vi "FTW-CodeGen-EnumerateVIServerClassHierarchy.vi"(0 "Class":string="GObject", 5 "Ancestor":string="Generic", 11 "error in":errorcluster) -> (6 "Is Descendent?":bool, 15 "error out":errorcluster)   [LabVIEW 2015]
panel:
  out "VI Server Class Hierarchy":T1(array[cluster])
  # "Inputs"
  # "Outputs"
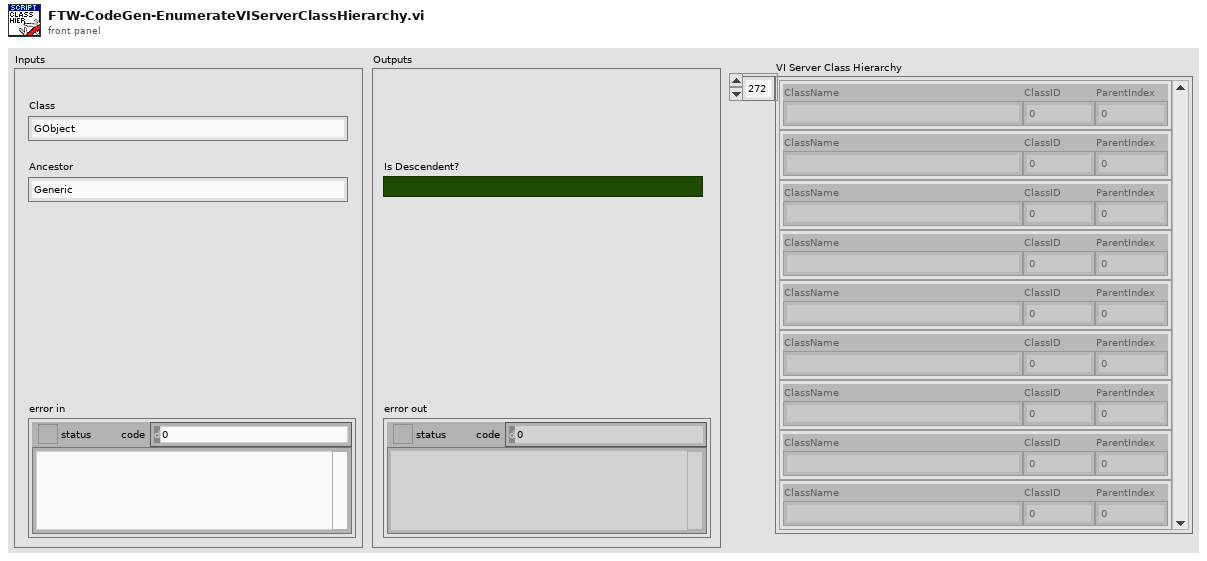
[diagram p1: front panel]
types:
  T1 = cluster{"ClassName":string, "ClassID":i32, "ParentIndex":i32}[]
  T2 = cluster{"ClassName":string, "ClassID":i32, "ParentIndex":i32}
  T3 = typedef "ASC_ArrayOfUniqueIDStringParentIDStringName.ctl" = T4[]
  T4 = typedef "ASC_UniqueIDStringParentIDStringName.ctl" = cluster{"Unique ID string":string, "Parent ID string":string, "Class Name (unlocalized)":string, "Class Name (localized)":string}
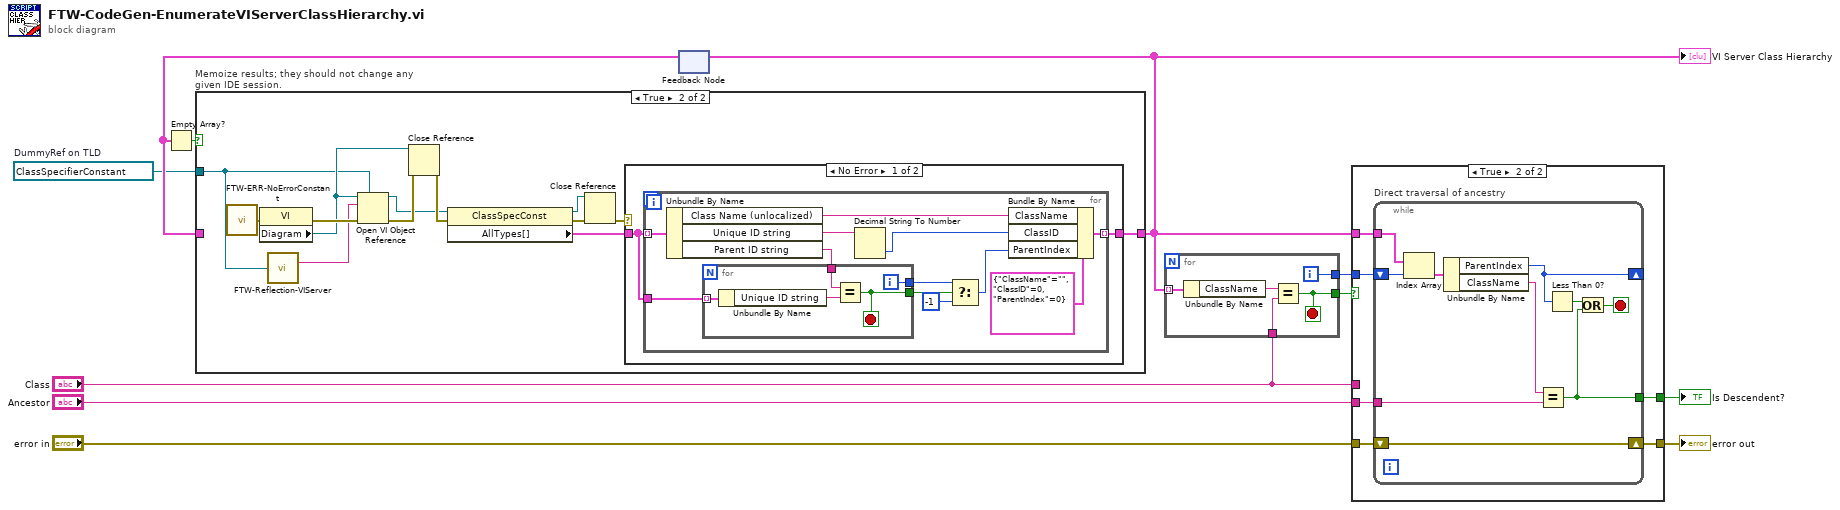
[diagram p0: block diagram]
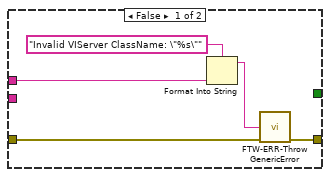
[diagram p2: hidden frame]
diagram:
  w9 = refnum<vi> refnum  # DummyRef on TLD
  n1 = feedback #1() -> (w11:T1)  [unwired: 1 in]
  n2 = Empty Array?(array=w11) -> (empty?=w10:bool)
  n3 = case "Memoize results; they should not change any given IDE session." shown="True" w10 {
    tunnel: [w12 w25] -> w4
    tunnel: w11 -> [w12 _]
    tunnel: w9 -> [_ w17]
    frame False {
    }
    frame True {
      n4 = call "FTW-ERR-NoErrorConstant.vi"() -> ("no error"=w14:errorcluster)
      n5 = property class="VI"(error in=w14) -> (error out=w24:errorcluster, "Diagram"=w21:refnum<vi>)  [unwired: 1 in, 1 out]
      n6 = call "FTW-Reflection-VIServer.vi"("VI Server Reference"=w17) -> ("Data Name"=w16:string)  [unwired: 11 in, 3 out]
      n7 = Open VI Object Reference(7:w17, 8:w24, 10:w16, 11:w21) -> (0:w23:errorcluster, 3:w20:refnum<vi>)
      n8 = Close Reference(reference=w21, error in (no error)=w23) -> (error out=w22:errorcluster)
      n9 = property class="ClassSpecConst"(reference=w20, error in=w22) -> (reference out=w18:refnum<vi>, error out=w19:errorcluster, "AllTypes[]"=w15:T3)
      n10 = Close Reference(reference=w18, error in (no error)=w19) -> (error out=w13:errorcluster)
      n11 = case shown="No Error" w13 {
        tunnel: [w27 _] -> w25
        tunnel: w15 -> [w26 _]
        frame No Error {
          n12 = for {
            tunnel: w26 -> [w39] mode=indexing
            tunnel: [w38] -> w27 mode=indexing
            tunnel: w26 -> [w34]
            n13 = Unbundle By Name(w39) -> ("Class Name (unlocalized)"=w37:string, "Unique ID string"=w36:string, "Parent ID string"=w33:string)
            n14 = for {
              tunnel: w34 -> [w44] mode=indexing
              tunnel: w33 -> [w43]
              tunnel: [w41] -> w32
              tunnel: [w40] -> w31
              i -> [w41]
              stop <- w40 stop-if-true
              n15 = Unbundle By Name(w44) -> ("Unique ID string"=w42:string)
              n16 = Equal?(x=w43, y=w42) -> (x = y?=w40:bool)
            }
            n17 = Decimal String To Number(string=w36) -> (number=w35:i32)  [unwired: 2 in, 1 out]
            n18 = Select(t=w32, s=w31, f=-1) -> (s? t:f=w30:i32)
            n19 = Bundle By Name(cluster=T2 {"ClassName"="", "ClassID"=0, "ParentIndex"=0}, "ClassName"=w37, "ClassID"=w35, "ParentIndex"=w30) -> (w38:T2)
          }
        }
        frame Error {
        }
      }
    }
  }
  "VI Server Class Hierarchy" <- w4
  n20 = feedback-in #1(w4) -> ()
  n21 = for {
    tunnel: "Class" -> [w47]
    tunnel: w4 -> [w49] mode=indexing
    tunnel: [w46] -> w5
    tunnel: [w45] -> w3
    i -> [w45]
    stop <- w46 stop-if-true
    n22 = Unbundle By Name(w49) -> ("ClassName"=w48:string)
    n23 = Equal?(x=w48, y=w47) -> (x = y?=w46:bool)
  }
  n24 = case shown="True" w5 {
    tunnel: "error in" -> [w54 w60]
    tunnel: [w53 w59] -> w7
    tunnel: "Ancestor" -> [_ w58]
    tunnel: w4 -> [_ w55]
    tunnel: w3 -> [_ w57]
    tunnel: "Class" -> [w50 _]
    tunnel: [_ w56] -> w1
    frame False {
      n25 = Format Into String(format string="Invalid VIServer ClassName: \"%s\"" ("Error Message"), w50) -> (resulting string=w51:string)  [unwired: 2 in, 1 out]
      n26 = call "FTW-ERR-ThrowGenericError.vi"("Error Message"=w51, "error in"=w54) -> ("error out"=w53:errorcluster)  [unwired: 13 in]
    }
    frame True {
      n27 = while "Direct traversal of ancestry" {
        shift-right: [w70] -> w59
        shift-left: w60 -> [w70]
        tunnel: w58 -> [w66]
        shift-right: [w65] -> _
        shift-left: w57 -> [w69]
        tunnel: [w62] -> w56
        tunnel: w55 -> [w61]
        stop <- w63 stop-if-true
        n28 = Index Array(array=w61, index=w69) -> (element=w68:T2)
        n29 = Unbundle By Name(w68) -> ("ParentIndex"=w65:i32, "ClassName"=w67:string)
        n30 = Equal?(x=w67, y=w66) -> (x = y?=w62:bool)
        n31 = Less Than 0?(x=w65) -> (x < 0?=w64:bool)
        n32 = Or(x=w64, y=w62) -> (x .or. y?=w63:bool)
      }
    }
  }
  "error out" <- w7
  "Is Descendent?" <- w1
